vi "Inject Attribute List.vi"(6 "Attributes Ref":refnum<data-value>, 8 "error in (no error)":errorcluster, 11 "Stop Bug Remover in":refnum<class "Stop Bug Remover.lvclass">) -> (0 "error out":errorcluster, 3 "Stop Bug Remover out":refnum<class "Stop Bug Remover.lvclass">)   [LabVIEW 2019, in "Stop Bug Remover.lvclass"]
uses:
  <vilib>/gpm_packages/@cs/Car-wash/Source/Process Steps/Stop Bug Remover/Stop Bug Remover.lvclass
  <vilib>/gpm_packages/@cs/lookup-table/Source/LookupTable/LookupTable.lvclass
  <vilib>/gpm_packages/@cs/lookup-table/Source/LookupTable/LookupTable.lvclass/LookupTable.ctl
  <vilib>/gpm_packages/@cs/Car-wash/Source/Process Steps/Stop Bug Remover/Stop Bug Remover.lvclass/Stop Bug Remover.ctl
  5bbc3a9f-15f3-4d1a-b5ba-4d112b6120bd.vi
  <vilib>/gpm_packages/@cs/lookup-table/Source/LookupTable/Read Table Reference.vi
  5bbc3a9f-15f3-4d1a-b5ba-4d112b6120bd.vi/8c43d355-d4aa-446c-aaf4-0d8522184eda.vi
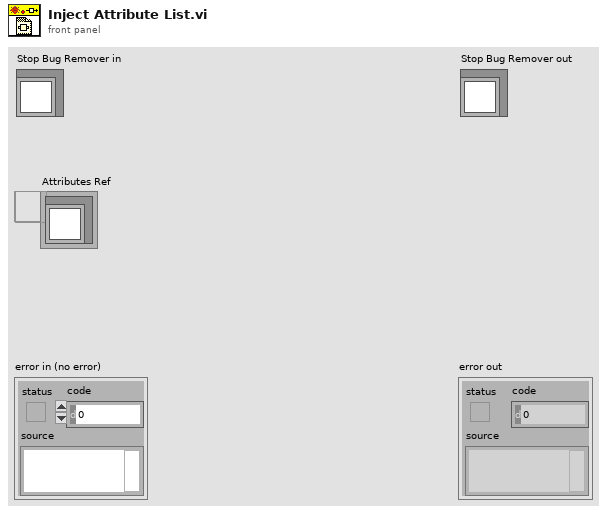
[diagram p1: front panel]
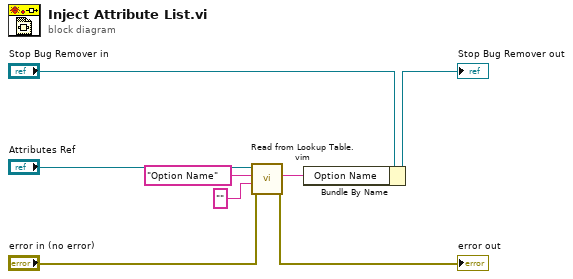
[diagram p0: block diagram]
diagram:
  n1 = call "Read from Lookup Table.vim"("error in (no error)"="error in (no error)", "Type"="", "Item Name"="Option Name", "LookupTable Reference"="Attributes Ref") -> ("error out"=→"error out":errorcluster, "Value"=w6:string)  [unwired: 4 in, 2 out]
  n2 = Bundle By Name(cluster="Stop Bug Remover in", "Option Name"=w6) -> (→"Stop Bug Remover out":refnum<class "Stop Bug Remover.lvclass">)
